vi "Start Acquisition.vi"(8 "error in (no error)":errorcluster, 11 "ImageHandler in":refnum<class "ImageHandler.lvclass">) -> (0 "error out":errorcluster, 2 "function return":i32, 3 "ImageHandler out":refnum<class "ImageHandler.lvclass">)   [LabVIEW 2022 SP3, in "ImageHandler.lvlib" / "ImageHandler.lvclass"]
uses:
  ImageHandler.lvclass
  BonTechDetector/Controls/Acquisition Commands.ctl
  ImageHandler.lvclass/ImageHandler.ctl
  BonTechDetector/BonTechDetector.lvlib
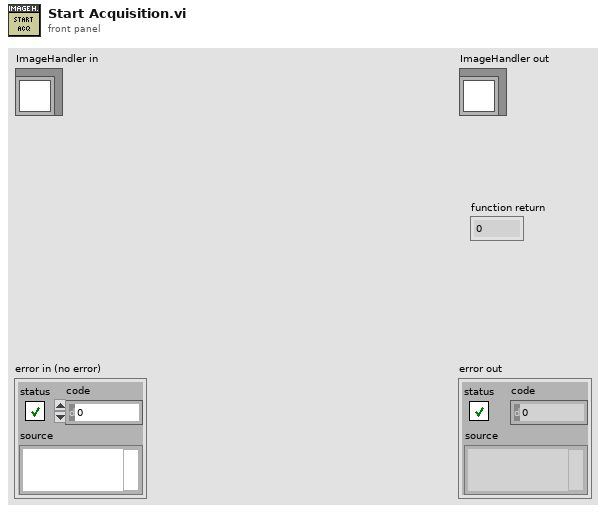
[diagram p1: front panel]
types:
  T1 = typedef "BonTechDetector.lvlib/Acquisition Commands.ctl" = u32
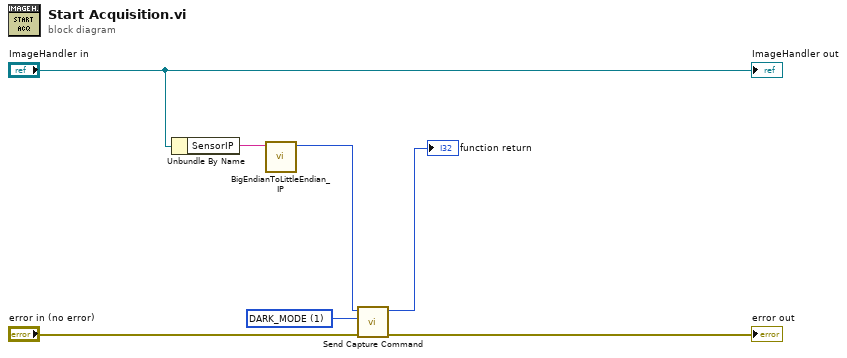
[diagram p0: block diagram]
diagram:
  w2 = T1 1 items=["ACQ_INIT"=0, "DARK_MODE"=1, "BRIGHT_MODE"=2, "SOFTTRIGGER_MODE"=258, "SOFTTRIGGER_INSTANT_MODE"=259] ("nCmd")
  n1 = Unbundle By Name("ImageHandler in") -> ("SensorIP"=w4:string)
  n2 = call "BigEndianToLittleEndian_IP.vi"("IP String"=w4) -> ("IP Network Order"=w3:u32)  [unwired: 10 in]
  n3 = call "Send Capture Command.vi"("error in (no error)"="error in (no error)", "nCmd"=w2, "nSensorIP"=w3) -> ("error out"=→"error out":errorcluster, "function return"=→"function return":i32)  [unwired: 7 in]
  "ImageHandler out" <- "ImageHandler in"
